vi "Update Tree Data's.vi"(7 "Data Cluster In":T2={"UI Reference"={"All Ctrl's Label's"=[], "ChannelListTree"=refnum, "All Object Ref"=[]}, "Tree Selection"={"Selected Channel"="", "Selected Interface"="", "Selected HW"="", "Tree Root Name"=""}, "Selected File Path"=path "", "Selected HW"={"Slctd Hw Name"=[], "Slctd HW IP"=[]}, "Channel Config Path"=path "", "Interface Data"={"DO Channel's"=[]}, "General Info's"={"Idnentification name"=""}, "Status"="", "Channel Type's"={"Channel Type"=enum."Voltage", "Sub-Type"=enum."Pressure"}, "This VI"=refnum, "Hardware Information "=variant(variant[] [])}, 8 "error in":errorcluster) -> (0 "error out":errorcluster, 5 "Data Cluster Out":T2={"UI Reference"={"All Ctrl's Label's"=[], "ChannelListTree"=refnum, "All Object Ref"=[]}, "Tree Selection"={"Selected Channel"="", "Selected Interface"="", "Selected HW"="", "Tree Root Name"=""}, "Selected File Path"=path "", "Selected HW"={"Slctd Hw Name"=[], "Slctd HW IP"=[]}, "Channel Config Path"=path "", "Interface Data"={"DO Channel's"=[]}, "General Info's"={"Idnentification name"=""}, "Status"="", "Channel Type's"={"Channel Type"=enum."Voltage", "Sub-Type"=enum."Pressure"}, "This VI"=refnum, "Hardware Information "=variant(variant[] [])})   [LabVIEW 2021, in "Configuration.lvlib"]
doc: "<b>Note:</b> This VI was modified by the <b>Validate DQMH Module</b> tool to turn off automatic error handling."
uses:
  Configuration.lvlib
  Module Data--cluster.ctl
  Host-Control's/Configuration UI Reference.ctl
  DO Channel's.ctl
  Config-Channel Type.ctl
  Channel Sub-Type.ctl
  Main Engine/Controls/Main Engine DAQ Device Info.ctl
  Main Engine/Controls/RT HW Info.ctl
  Main Engine/Controls/Main Engine Serial Info JSON Data.ctl
  Main Engine/Controls/Main Engine DAQ Harware Info JSON Data.ctl
  Main Engine/Controls/Main Engine Ehernet IP Address JSON Data.ctl
  <vilib>/Utility/miscctls.llb/LVMapReplaceAction.ctl
  <vilib>/National Instruments/Tree Map/API/List Roots.vi
  <vilib>/National Instruments/Tree Map/Utility/Into Tree Control Items.vi
  <vilib>/National Instruments/Tree Map/Tree Map.lvlib
panel:
  out "DAQ Device Info":T1[](array[typedef])
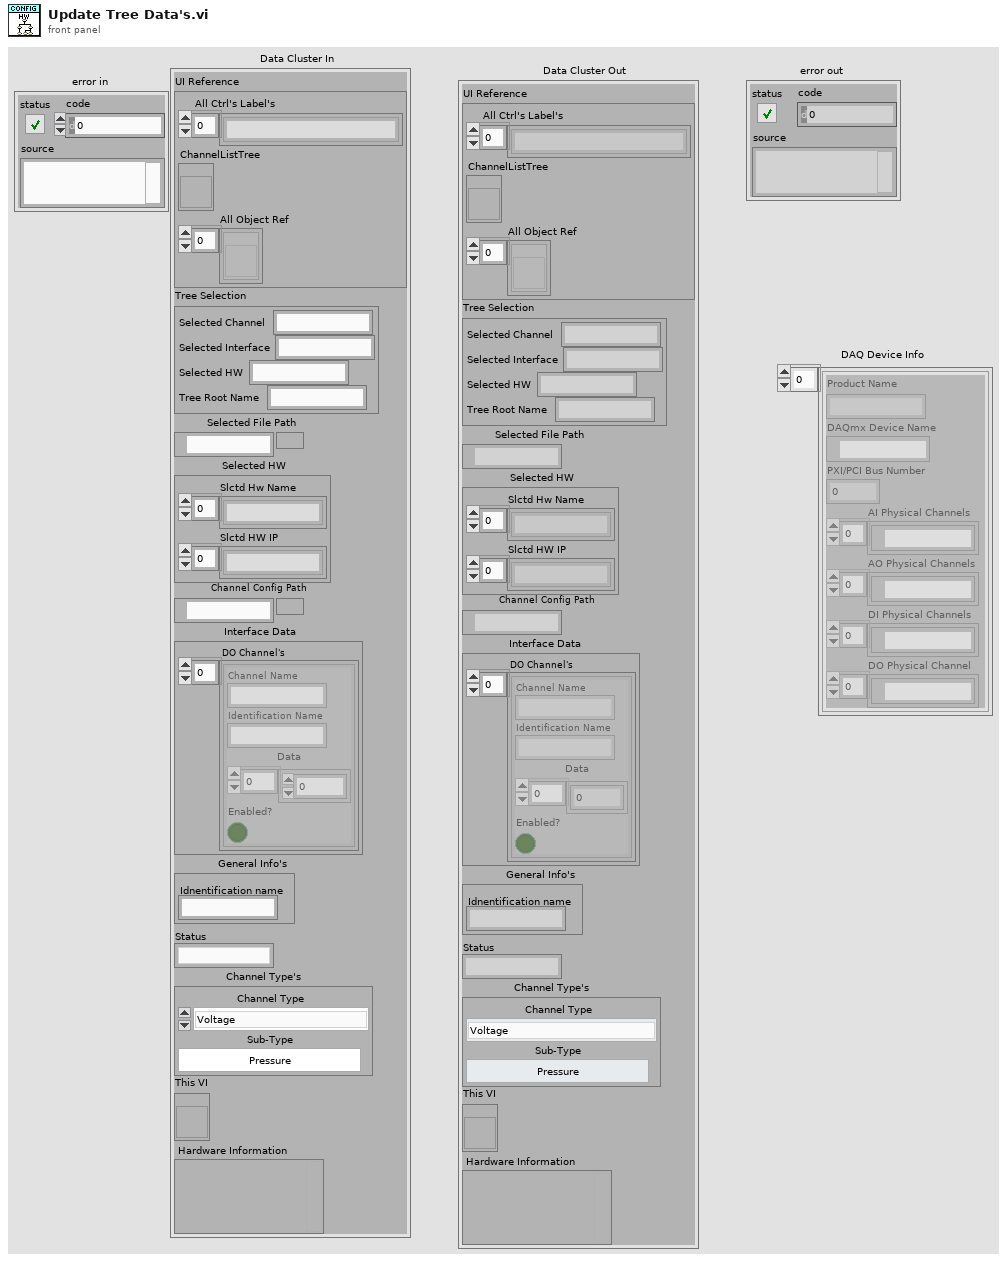
[diagram p1: front panel]
types:
  T1 = typedef "Main Engine DAQ Device Info.ctl" = cluster{"Product Name":string, "DAQmx Device Name":tag, "PXI/PCI Bus Number":u32, "AI Physical Channels":tag[], "AO Physical Channels":tag[], "DI Physical Channels":tag[], "DO Physical Channel":tag[]}
  T2 = typedef "Configuration.lvlib/Module Data--cluster.ctl" = cluster{"UI Reference":T3, "Tree Selection":cluster{"Selected Channel":string, "Selected Interface":string, "Selected HW":string, "Tree Root Name":string}, "Selected File Path":path, "Selected HW":cluster{"Slctd Hw Name":string[], "Slctd HW IP":string[]}, "Channel Config Path":path, "Interface Data":cluster{"DO Channel's":T4}, "General Info's":cluster{"Idnentification name":string}, "Status":string, "Channel Type's":cluster{"Channel Type":T5, "Sub-Type":T6}, "This VI":refnum<vi>, "Hardware Information ":variant}
  T3 = typedef "Configuration UI Reference.ctl" = cluster{"All Ctrl's Label's":string[], "ChannelListTree":refnum<vi>, "All Object Ref":refnum<vi>[]}
  T4 = typedef "Configuration.lvlib/DO Channel's.ctl" = cluster{"Channel Name":string, "Identification Name":string, "Data":u8[], "Enabled?":bool}[]
  T5 = typedef "Configuration.lvlib/Config-Channel Type.ctl" = enum16{"Voltage", "Current", "Thermocouple", "Acclerometer"}
  T6 = typedef "Configuration.lvlib/Channel Sub-Type.ctl" = enum16{"None", "Pressure", "Force"}
  T7 = cluster{"DAQ Device Info":T1[], "Ethernet IP Address":string[]}
  T8 = typedef "RT HW Info.ctl" = cluster{"Serial Hardware Info JSON Format":T9, "Analog HW Info JSON Format":T10, "Digital HW Info JSON Format":T10, "Ethernet IP Address JSON Format":T11}
  T9 = typedef "Main Engine Serial Info JSON Data.ctl" = cluster{"Command":string, "SubCmd":string, "Channel":string[]}
  T10 = typedef "Main Engine DAQ Harware Info JSON Data.ctl" = cluster{"Command":string, "SubCmd":string, "Input":string[], "Output":string[]}
  T11 = typedef "Main Engine Ehernet IP Address JSON Data.ctl" = cluster{"Command":string, "SubCmd":string, "IP":string[]}
  T12 = typedef "Tree Map.lvlib/Tree Map Data.ctl" = map{string, cluster{"Child Paths Set":set{string}, "Name":string, "Data":string, "Attributes":map{string, string}}}
  T13 = typedef "LVMapReplaceAction.ctl" = enum32{"Modify Entry only if found", "Add or Modify Entry", "Delete Entry"}
  T14 = cluster{"Left Cell String":string, "Child Text":string[], "Child Tag":string, "Item Indent":i32, "Child Only?":bool, "Glyph Index":i32}[]
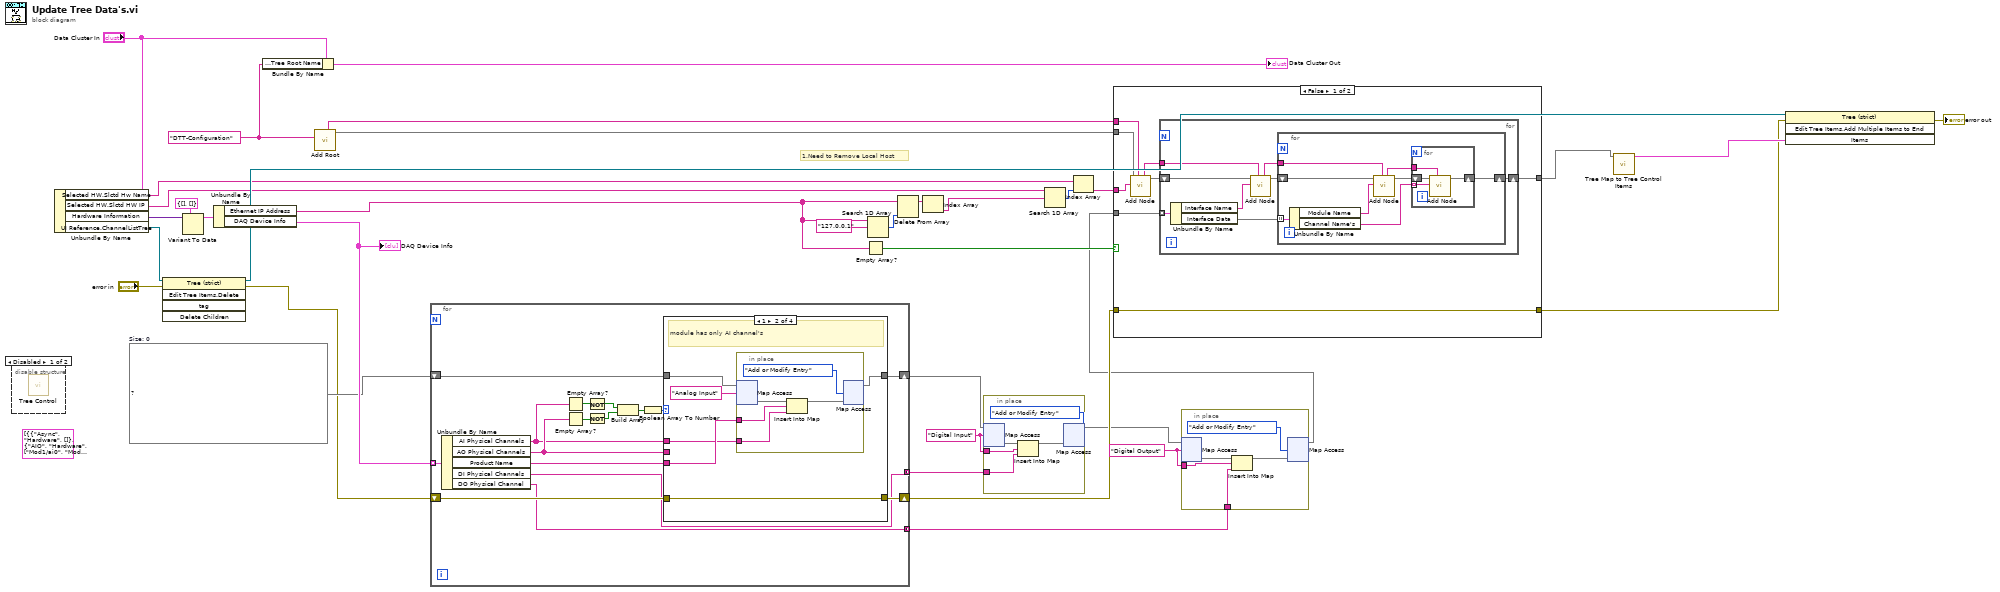
[diagram p0: block diagram]
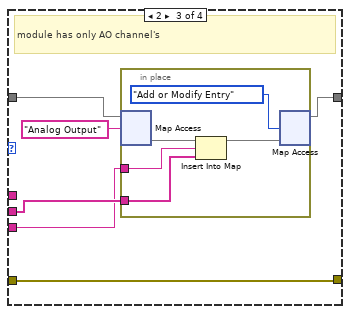
[diagram p3: hidden frame]
diagram:
  w3 = "Digital Output" ("New Node Name")
  w6 = "Digital Input" ("New Node Name")
  w10 = map{string, map{string, string[]}} {}  # Size: 0
  (unwired) T8[] [{"Serial Hardware Info JSON Format"={"Command"="Async", "SubCmd"="Hardware", "Channel"=[]}, "Analog HW Info JSON Format"={"Command"="AIO", "SubCmd"="Hardware", "Input"=["Mod1/ai0", "Mod1/ai1", "Mod1/ai2", "Mod1/ai3", "Mod3/ai0", "Mod3/ai1", "Mod3/ai2", "Mod3/ai3", "Mod3/ai4", "Mod3/ai5", "Mod3/ai6", "Mod3/ai7", "Mod3/ai8", "Mod3/ai9", "Mod3/ai10", "Mod3/ai11", "Mod3/ai12", "Mod3/ai13", "Mod3/ai14", "Mod3/ai15", "Mod8/ai0", "Mod8/ai1", "Mod8/ai2", "Mod8/ai3", "Mod8/ai4", "Mod8/ai5", "Mod8/ai6", "Mod8/ai7", "Mod8/ai8", "Mod8/ai9", "Mod8/ai10", "Mod8/ai11", "Mod8/ai12", "Mod8/ai13", "Mod8/ai14", "Mod8/ai15"], "Output"=["Mod2/ao0", "Mod2/ao1", "Mod2/ao2", "Mod2/ao3", "Mod2/ao4", "Mod2/ao5", "Mod2/ao6", "Mod2/ao7", "Mod2/ao8", "Mod2/ao9", "Mod2/ao10", "Mod2/ao11", "Mod2/ao12", "Mod2/ao13", "Mod2/ao14", "Mod2/ao15"]}, "Digital HW Info JSON Format"={"Command"="DIO", "SubCmd"="Hardware", "Input"=["Mod5/port0/line0", "Mod5/port0/line1", "Mod5/port0/line2", "Mod5/port0/line3", "Mod5/port0/line4", "Mod5/port0/line5", "Mod5/port0/line6", "Mod5/port0/line7", "Mod6/port0/line0", "Mod6/port0/line1", "Mod6/port0/line2", "Mod6/port0/line3", "Mod6/port0/line4", "Mod6/port0/line5", "Mod6/port0/line6", "Mod6/port0/line7", "Mod6/port0/line8", "Mod6/port0/line9", "Mod6/port0/line10", "Mod6/port0/line11", "Mod6/port0/line12", "Mod6/port0/line13", "Mod6/port0/line14", "Mod6/port0/line15"], "Output"=["Mod5/port0/line0", "Mod5/port0/line1", "Mod5/port0/line2", "Mod5/port0/line3", "Mod5/port0/line4", "Mod5/port0/line5", "Mod5/port0/line6", "Mod5/port0/line7", "Mod6/port1/line0", "Mod6/port1/line1", "Mod6/port1/line2", "Mod6/port1/line3", "Mod6/port1/line4", "Mod6/port1/line5", "Mod6/port1/line6", "Mod6/port1/line7", "Mod6/port1/line8", "Mod6/port1/line9", "Mod6/port1/line10", "Mod6/port1/line11", "Mod6/port1/line12", "Mod6/port1/line13", "Mod6/port1/line14", "Mod6/port1/line15"]}, "Ethernet IP Address JSON Format"={"Command"="Ethernet", "SubCmd"="Hardware", "IP"=["192.168.32.50", "127.0.0.1"]}}, {"Serial Hardware Info JSON Format"={"Command"="", "SubCmd"="", "Channel"=[]}, "Analog HW Info JSON Format"={"Command"="", "SubCmd"="", "Input"=[], "Output"=[]}, "Digital HW Info JSON Format"={"Command"="", "SubCmd"="", "Input"=[], "Output"=[]}, "Ethernet IP Address JSON Format"={"Command"="", "SubCmd"="", "IP"=[]}}] ("RT HW Info 2")
  w22 = "DTT-Configuration" ("New Root Name")
  # "1.Need to Remove Local Host"
  n1 = disable-structure shown="Disabled" {
    frame Disabled {
      n2 = call <vilib>:"Tree Control.vi"() -> ()  [unwired: 12 in]
    }
    frame Enabled {
    }
  }
  n3 = Unbundle By Name("Data Cluster In") -> ("Selected HW.Slctd Hw Name"=w25:string[], "Selected HW.Slctd HW IP"=w26:string[], "Hardware Information"=w27:variant, "UI Reference.ChannelListTree"=w28:refnum<vi>)
  n4 = invoke class="Tree (strict)" method="Edit Tree Items.Delete"(reference=w28, error in="error in") -> (reference out=w31:refnum<vi>, error out=w8:errorcluster)  [unwired: 3 in, 3 out]
  n5 = Variant To Data(type=T7 {"DAQ Device Info"=[], "Ethernet IP Address"=[]} ("output cluster"), Variant=w27) -> (data=w13:T7)  [unwired: 1 in, 1 out]
  n6 = Unbundle By Name(w13) -> ("Ethernet IP Address"=w12:string[], "DAQ Device Info"=w11:T1[])
  "DAQ Device Info" <- w11
  n7 = Bundle By Name(cluster="Data Cluster In", "Tree Selection.Tree Root Name"=w22) -> (→"Data Cluster Out":T2)
  n8 = call <vilib>:"Add Root.vi"("New Root Name"=w22) -> ("Tree Map Out"=w33:T12, "Root Path"=w34:string)  [unwired: 9 in]
  n9 = for {
    tunnel: w11 -> [w52] mode=indexing
    shift-right: [w41] -> w7
    shift-left: w10 -> [w42]
    shift-right: [w40] -> w9
    shift-left: w8 -> [w39]
    tunnel: [w38] -> w5 mode=concatenating
    tunnel: [w37] -> w2 mode=concatenating
    n10 = Unbundle By Name(w52) -> ("AI Physical Channels"=w43:tag[], "AO Physical Channels"=w44:tag[], "Product Name"=w45:string, "DI Physical Channels"=w38:tag[], "DO Physical Channel"=w37:tag[])
    n11 = Empty Array?(array=w43) -> (empty?=w51:bool)
    n12 = Empty Array?(array=w44) -> (empty?=w50:bool)
    n13 = Not(x=w51) -> (.not. x?=w49:bool)
    n14 = Not(x=w50) -> (.not. x?=w48:bool)
    n15 = Build Array(w49, w48) -> (w47:bool[])
    n16 = Boolean Array To Number(Boolean array=w47) -> (number=w46:u32)
    n17 = case shown="1" w46 {
      tunnel: w45 -> [_ w58 w68 _]
      tunnel: w44 -> [_ _ w69 _]
      tunnel: w43 -> [_ w55 _ _]
      tunnel: w42 -> [w54 w60 w71 w78]
      tunnel: [w54 w57 w67 w78] -> w41
      tunnel: [w53 w56 w66 w77] -> w40
      tunnel: w39 -> [w53 w56 w66 w77]
      frame 0, Default {
        # "All are False i.e module has no AI,AO,DI,DO channel's"
      }
      frame 1 {
        # "module has only AI channel's"
        n18 = in-place {
          in-place-border: w58 -> [w64]
          in-place-border: w55 -> [w63]
          n19 = in-place-map #1(w60, "Analog Input" ("New Node Name")) -> (w65:map{string, string[]})  [unwired: 1 in, 1 out]
          n20 = Insert Into Map(map in=w65, key=w64, value=w63) -> (map out=w62:map{string, string[]})  [unwired: 2 out]
          n21 = in-place-map #1(w62, LVMapReplaceAction."Add or Modify Entry" ("action")) -> (w57:map{string, map{string, string[]}})  [unwired: 2 out]
        }
      }
      frame 2 {
        # "module has only AO channel's"
        n22 = in-place {
          in-place-border: w68 -> [w75]
          in-place-border: w69 -> [w74]
          n23 = in-place-map #2(w71, "Analog Output" ("New Node Name")) -> (w76:map{string, string[]})  [unwired: 1 in, 1 out]
          n24 = Insert Into Map(map in=w76, key=w75, value=w74) -> (map out=w73:map{string, string[]})  [unwired: 2 out]
          n25 = in-place-map #2(w73, LVMapReplaceAction."Add or Modify Entry" ("action")) -> (w67:map{string, map{string, string[]}})  [unwired: 2 out]
        }
      }
      frame 3 {
        # "module has both AI and  AO channel's"
      }
    }
  }
  n26 = Empty Array?(array=w12) -> (empty?=w15:bool)
  n27 = Search 1D Array(1D array=w12, element="127.0.0.1") -> (index of element=w20:i32)  [unwired: 1 in]
  n28 = Delete From Array(array=w12, index=w20) -> (array with subset deleted=w19:string[])  [unwired: 1 in, 1 out]
  n29 = Index Array(array=w19) -> (element=w18:string)  [unwired: 1 in]
  n30 = in-place {
    in-place-border: w6 -> [w81]
    in-place-border: w5 -> [w80]
    n31 = in-place-map #3(w7, w6) -> (w82:map{string, string[]})  [unwired: 1 in, 1 out]
    n32 = Insert Into Map(map in=w82, key=w81, value=w80) -> (map out=w79:map{string, string[]})  [unwired: 2 out]
    n33 = in-place-map #3(w79, LVMapReplaceAction."Add or Modify Entry" ("action")) -> (w4:map{string, map{string, string[]}})  [unwired: 2 out]
  }
  n34 = Search 1D Array(1D array=w26, element=w18) -> (index of element=w17:i32)  [unwired: 1 in]
  n35 = Index Array(array=w25, index=w17) -> (element=w16:string)
  n36 = in-place {
    in-place-border: w3 -> [w86]
    in-place-border: w2 -> [w85]
    n37 = in-place-map #4(w4, w3) -> (w87:map{string, string[]})  [unwired: 1 in, 1 out]
    n38 = Insert Into Map(map in=w87, key=w86, value=w85) -> (map out=w84:map{string, string[]})  [unwired: 2 out]
    n39 = in-place-map #4(w84, LVMapReplaceAction."Add or Modify Entry" ("action")) -> (w1:map{string, map{string, string[]}})  [unwired: 2 out]
  }
  n40 = case shown="False" w15 {
    tunnel: w34 -> [w96 _]
    tunnel: w33 -> [w95 w117]
    tunnel: [w89 w117] -> w35
    tunnel: w16 -> [w94 _]
    tunnel: [w93 w118] -> w30
    tunnel: w9 -> [w93 w118]
    tunnel: w1 -> [w92 _]
    frame False {
      n41 = call <vilib>:"Add Node.vi"("Parent Path"=w96, "New Node Name"=w94, "Tree Map In"=w95) -> ("Tree Map Out"=w91:T12, "New Node Path"=w90:string)  [unwired: 6 in, 1 out]
      n42 = for {
        tunnel: w92 -> [w104] mode=indexing
        shift-right: [w97] -> w89
        shift-left: w91 -> [w103]
        tunnel: w90 -> [w101]
        n43 = Unbundle By Name(w104) -> ("Interface Name"=w102:string, "Interface Data"=w100:map{string, string[]})
        n44 = call <vilib>:"Add Node.vi"("Parent Path"=w101, "New Node Name"=w102, "Tree Map In"=w103) -> ("Tree Map Out"=w99:T12, "New Node Path"=w98:string)  [unwired: 6 in, 1 out]
        n45 = for {
          tunnel: w100 -> [w112] mode=indexing
          tunnel: w98 -> [w110]
          shift-right: [w105] -> w97
          shift-left: w99 -> [w111]
          n46 = Unbundle By Name(w112) -> ("Module Name"=w109:string, "Channel Name's"=w106:string[])
          n47 = call <vilib>:"Add Node.vi"("Parent Path"=w110, "New Node Name"=w109, "Tree Map In"=w111) -> ("Tree Map Out"=w108:T12, "New Node Path"=w107:string)  [unwired: 6 in, 1 out]
          n48 = for {
            shift-right: [w116] -> w105
            shift-left: w108 -> [w113]
            tunnel: w106 -> [w115] mode=indexing
            tunnel: w107 -> [w114]
            n49 = call <vilib>:"Add Node.vi"("Parent Path"=w114, "New Node Name"=w115, "Tree Map In"=w113) -> ("Tree Map Out"=w116:T12)  [unwired: 6 in, 2 out]
          }
        }
      }
    }
    frame True {
    }
  }
  n50 = call <vilib>:"Tree Map to Tree Control Items.vi"("Tree Map In"=w35) -> ("Tree Control Items"=w36:T14)  [unwired: 10 in]
  n51 = invoke class="Tree (strict)" method="Edit Tree Items.Add Multiple Items to End"(reference=w31, error in=w30, "Items"=w36) -> (error out=→"error out":errorcluster)  [unwired: 1 in, 3 out]
